vi "Command RPED Left.vi"(11 "Startup":bool) -> (2 "RPED Left":dbl, 4 "Reinit":bool, 5 "Completed":bool)   [LabVIEW 2017]
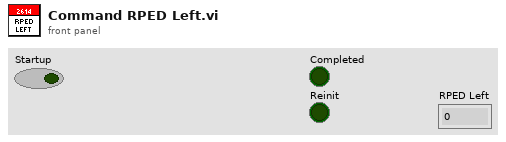
[diagram p1: front panel]
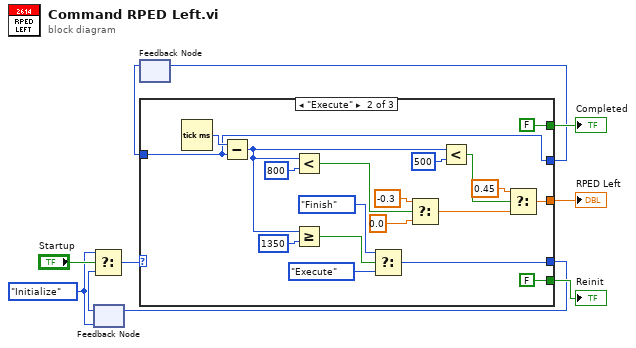
[diagram p0: block diagram]
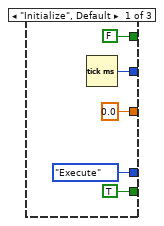
[diagram p2: hidden frame]
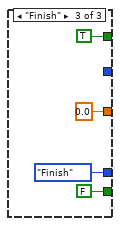
[diagram p3: hidden frame]
diagram:
  w8 = enum16{"Initialize", "Execute", "Finish"}."Initialize"
  n1 = feedback #1(w8) -> (w3:enum16{"Initialize", "Execute", "Finish"})
  n2 = Select(t=w8, s="Startup", f=w3) -> (s? t:f=w9:enum16{"Initialize", "Execute", "Finish"})
  n3 = feedback #2() -> (w2:u32)  [unwired: 1 in]
  n4 = case shown="\"Execute\"" w9 {
    tunnel: [FALSE FALSE TRUE] -> w7
    tunnel: [TRUE FALSE FALSE] -> w6
    tunnel: [enum16{"Initialize", "Execute", "Finish"}."Execute" w19 enum16{"Initialize", "Execute", "Finish"}."Finish"] -> w5
    tunnel: [w12 w31 _] -> w4
    tunnel: w2 -> [_ w31 _]
    tunnel: [0.0 ("Left Wheel Velocity") w28 0.0] -> w1
    frame "Initialize", Default {
      n5 = Tick Count (ms)() -> (millisecond timer value=w12:u32)
    }
    frame "Execute" {
      n6 = Tick Count (ms)() -> (millisecond timer value=w34:u32)
      n7 = Subtract(x=w34, y=w31) -> (x-y=w21:u32)
      n8 = Less?(x=w21, y=u32 800) -> (x < y?=w25:bool)
      n9 = Greater Or Equal?(x=w21, y=u32 1350) -> (x >= y?=w18:bool)
      n10 = Select(t=enum16{"Initialize", "Execute", "Finish"}."Finish", s=w18, f=enum16{"Initialize", "Execute", "Finish"}."Execute") -> (s? t:f=w19:enum16{"Initialize", "Execute", "Finish"})
      n11 = Select(t=-0.3, s=w25, f=0.0) -> (s? t:f=w26:dbl)
      n12 = Less?(x=w21, y=u32 500) -> (x < y?=w29:bool)
      n13 = Select(t=0.45, s=w29, f=w26) -> (s? t:f=w28:dbl)
    }
    frame "Finish" {
    }
  }
  "Completed" <- w7
  "Reinit" <- w6
  "RPED Left" <- w1
  n14 = feedback-in #1(w5) -> ()
  n15 = feedback-in #2(w4) -> ()
